vi "Calc_Average_Counts.vi"(0 "Mode":enum16{"Initialize", "Accumulate"}(ring), 2 "NumPixels":i32, 3 "Spectra":dbl[](array[numeric]), 5 "Pressure in":dbl, 6 "Temperature in":dbl, 7 "error in":errorcluster, 8 "State in":i32, 10 "Calculation config data":T1) -> (9 "First?":bool, 12 "Pressure during R":dbl, 14 "Temperature during R":dbl, 16 "R counts":dbl[](array[numeric]), 18 "Zero counts":dbl[](array[numeric]), 19 "Calc R?":bool, 20 "Ch1 Dark":dbl[](array[numeric]), 21 "Pressure during Zero":dbl, 22 "Temperature during Zero":dbl, 27 "error out":errorcluster)   [LabVIEW 2025]
uses:
  Configuration/TypeDef_CalculationConfigData.ctl
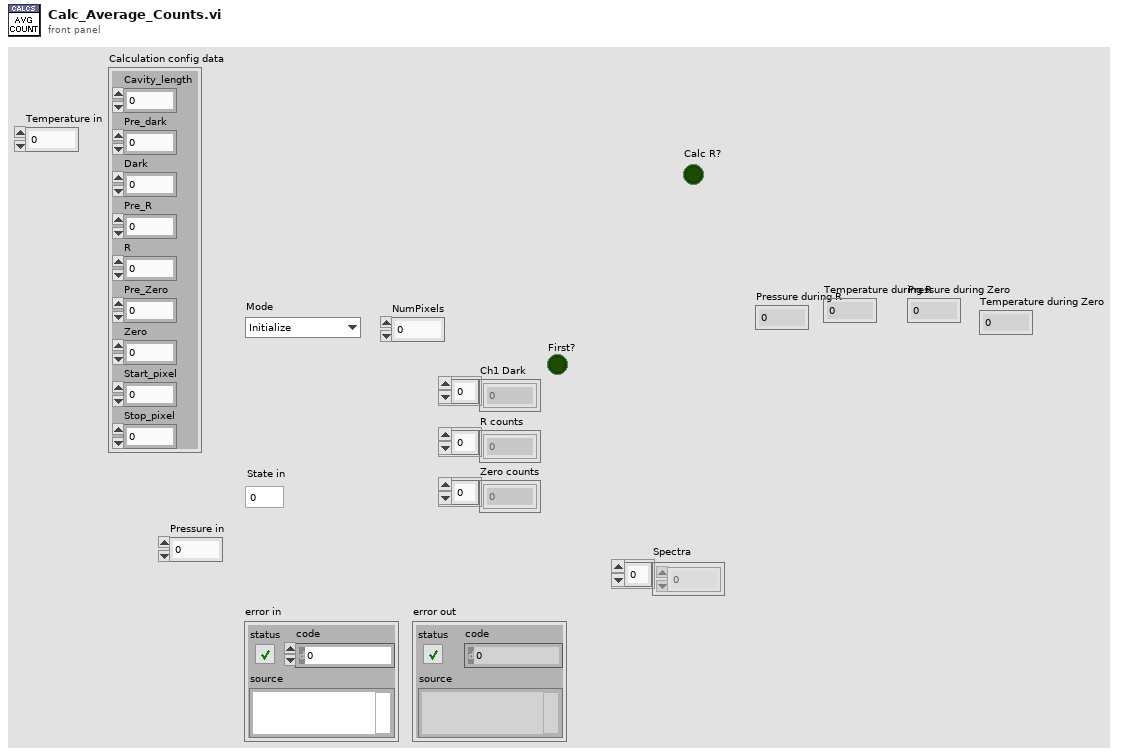
[diagram p1: front panel]
types:
  T1 = typedef "TypeDef_CalculationConfigData.ctl" = cluster{"Cavity_length":dbl, "Pre_dark":i32, "Dark":i32, "Pre_R":i32, "R":i32, "Pre_Zero":i32, "Zero":i32, "Start_pixel":i32, "Stop_pixel":i32}
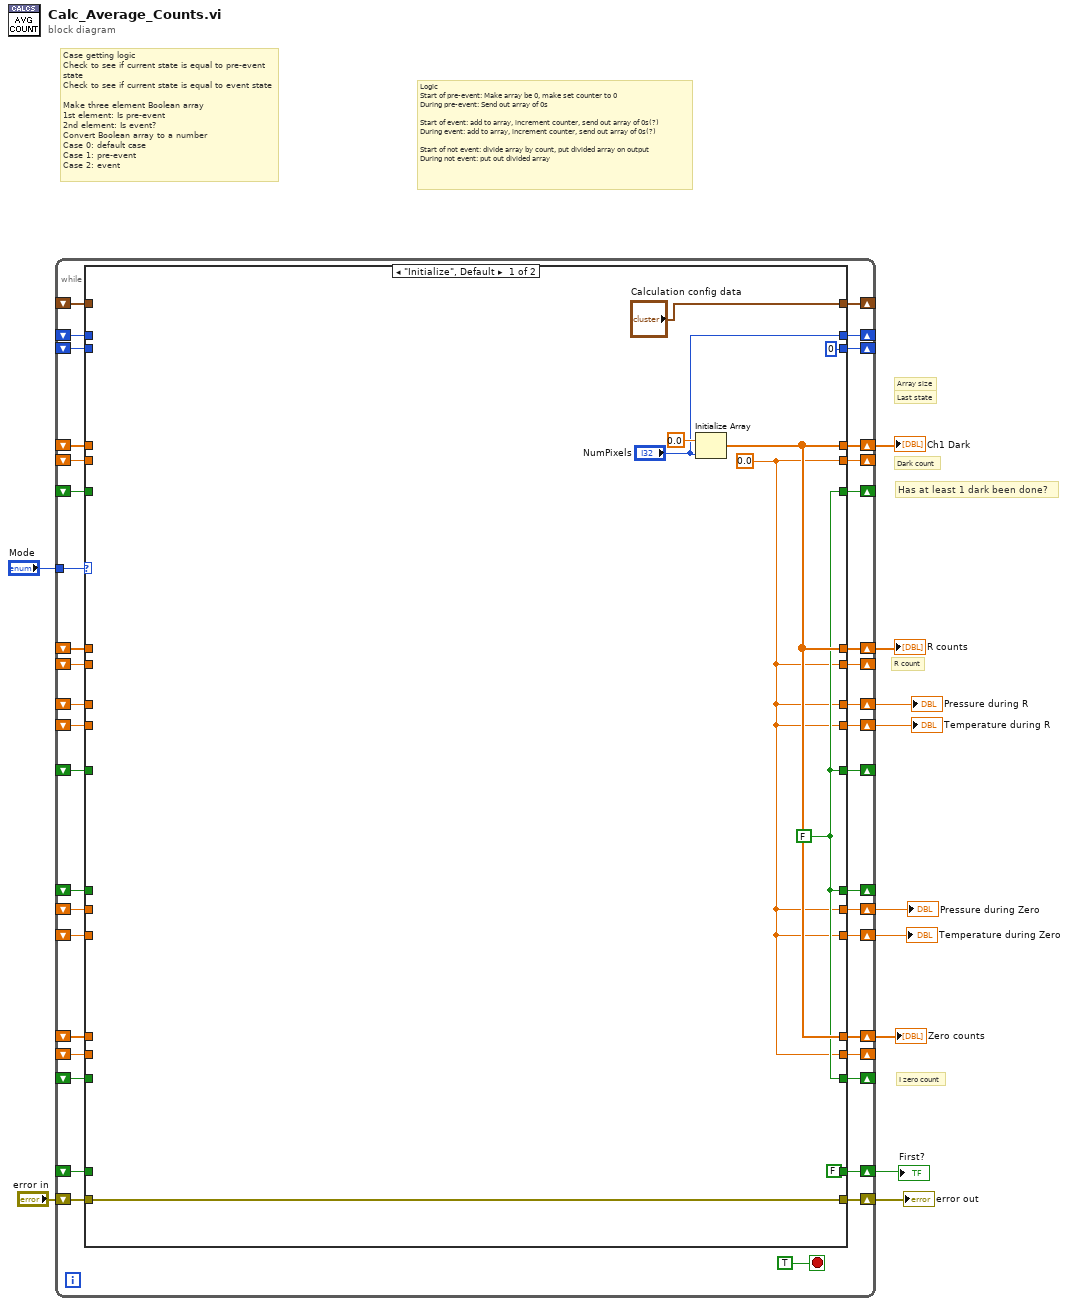
[diagram p0: block diagram]
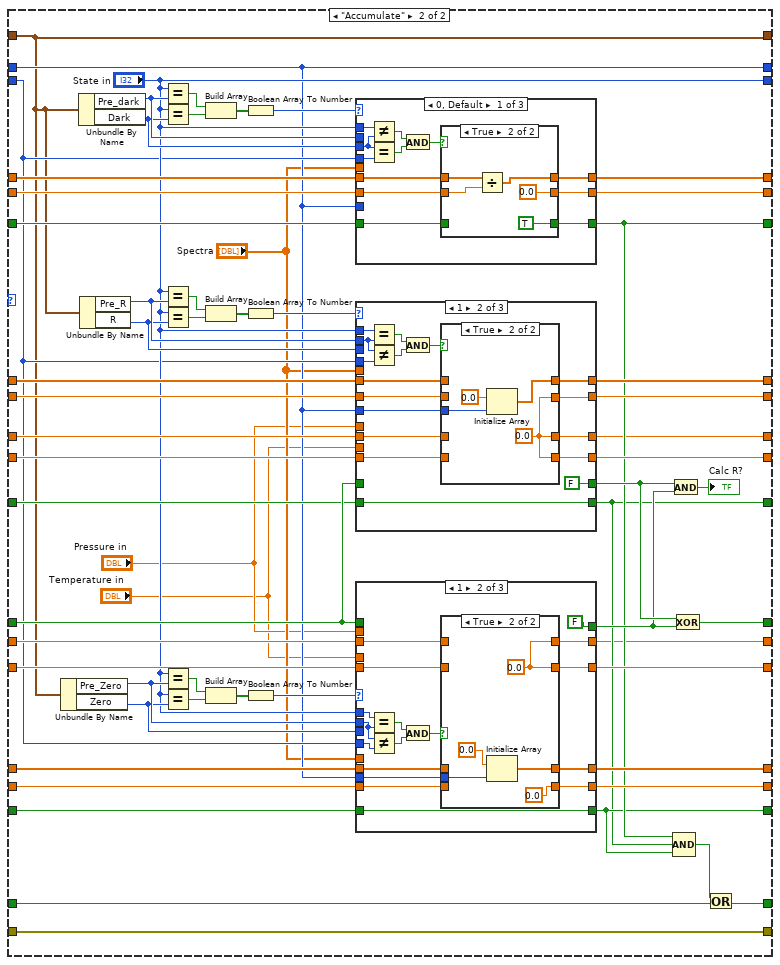
[diagram p2: hidden frame]
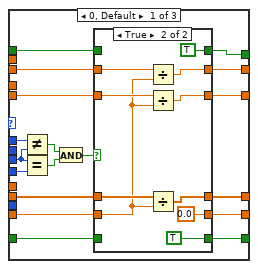
[diagram p3: hidden frame]
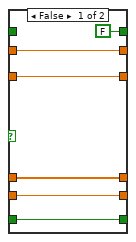
[diagram p4: hidden frame]
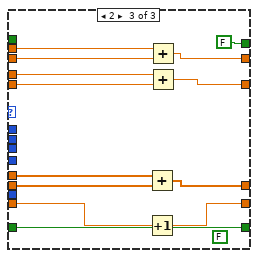
[diagram p6: hidden frame]
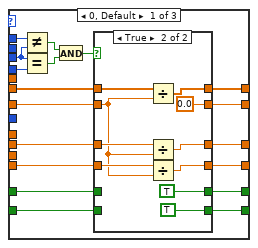
[diagram p7: hidden frame]
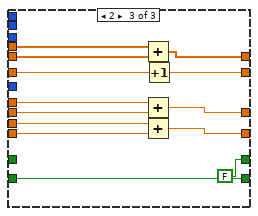
[diagram p10: hidden frame]
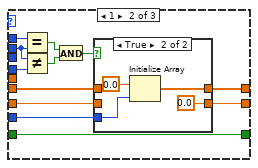
[diagram p12: hidden frame]
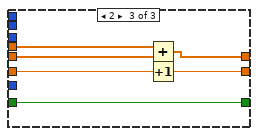
[diagram p14: hidden frame]
diagram:
  # "Has at least 1 dark been done?"
  # "Case getting logic\nCheck to see if current state is equal to pre-event state\nCheck to see if current state is equal to event state\n\nMake three element Boolean array \n1st element: Is pre-event\n2nd element: Is event?\nConvert Boolean array to a number\nCase 0: default case\nCase 1: pre-event\nCase 2: event"
  # "Logic\nStart of pre-event: Make array be 0, make set counter to 0\nDuring pre-event: Send out array of 0s\n\nStart of event: add to array, increment counter, send out array of 0s(?)\nDuring event: add to array, increment counter, send out array of 0s(?)\n\nStart of not event: divide array by count, put divided array on output\nDuring not event: put out divided array"
  # "Array size"
  # "Last state"
  # "I zero count"
  # "R count"
  # "Dark count"
  n1 = while {
    tunnel: "Mode" -> [w50]
    shift-right: [w48] -> w9
    shift-left: "error in" -> [w49]
    shift-right: [w47] -> w8
    shift-left: _ -> [w46]
    shift-right: [w45] -> _
    shift-left: _ -> [w34]
    shift-right: [w44] -> w7
    shift-left: _ -> [w42]
    shift-right: [w43] -> w6
    shift-left: _ -> [w41]
    shift-right: [w40] -> _
    shift-left: _ -> [w37]
    shift-right: [w39] -> _
    shift-left: _ -> [w38]
    shift-right: [w36] -> _
    shift-left: _ -> [w35]
    shift-right: [w33] -> _
    shift-left: _ -> [w32]
    shift-right: [w14] -> w2
    shift-left: _ -> [w28]
    shift-right: [w31] -> w1
    shift-left: _ -> [w27]
    shift-right: [w29] -> w4
    shift-left: _ -> [w26]
    shift-right: [w30] -> w3
    shift-left: _ -> [w25]
    shift-right: [w24] -> _
    shift-left: _ -> [w23]
    shift-right: [w22] -> w5
    shift-left: _ -> [w21]
    shift-right: [w20] -> _
    shift-left: _ -> [w16]
    shift-right: [w19] -> _
    shift-left: _ -> [w15]
    shift-right: [w18] -> _
    shift-left: _ -> [w17]
    shift-right: [w13] -> _
    shift-left: _ -> [w12]
    stop <- TRUE stop-if-true
    n2 = case shown="\"Initialize\", Default" w50 {
      tunnel: w49 -> [w60 w120]
      tunnel: [w60 w120] -> w48
      tunnel: [w56 w113] -> w47
      tunnel: w46 -> [_ w115]
      tunnel: [w53 w112] -> w45
      tunnel: [w56 w105] -> w44
      tunnel: [w56 w97] -> w43
      tunnel: w42 -> [_ w106]
      tunnel: w41 -> [_ w99]
      tunnel: [w53 w103] -> w40
      tunnel: [w53 w96] -> w39
      tunnel: w38 -> [_ w98]
      tunnel: w37 -> [_ w104]
      tunnel: [0 ("dimension size") "State in"] -> w36
      tunnel: w35 -> [_ w69]
      tunnel: w34 -> [_ w114]
      tunnel: ["NumPixels" w68] -> w33
      tunnel: w32 -> [_ w68]
      tunnel: [w53 w63] -> w14
      tunnel: [w53 w87] -> w31
      tunnel: [w53 w84] -> w30
      tunnel: [w53 w67] -> w29
      tunnel: w28 -> [_ w89]
      tunnel: w27 -> [_ w88]
      tunnel: w26 -> [_ w86]
      tunnel: w25 -> [_ w85]
      tunnel: [w54 w83] -> w24
      tunnel: w23 -> [_ w80]
      tunnel: [FALSE w77] -> w22
      tunnel: w21 -> [_ w78]
      tunnel: [w54 w76] -> w20
      tunnel: [w54 w72] -> w19
      tunnel: [w54 w73] -> w18
      tunnel: w17 -> [_ w74]
      tunnel: w16 -> [_ w75]
      tunnel: w15 -> [_ w71]
      tunnel: ["Calculation config data" w61] -> w13
      tunnel: w12 -> [_ w61]
      frame "Initialize", Default {
        w54 = FALSE
        w53 = 0.0 ("dimension size")
        n3 = Initialize Array(0.0 ("element"), "NumPixels") -> (w56:dbl[])
      }
      frame "Accumulate" {
        n4 = Unbundle By Name(w61) -> ("Pre_Zero"=w91:i32, "Zero"=w90:i32)
        n5 = Unbundle By Name(w61) -> ("Pre_dark"=w111:i32, "Dark"=w110:i32)
        n6 = Unbundle By Name(w61) -> ("Pre_R"=w101:i32, "R"=w100:i32)
        n7 = Equal?(x="State in", y=w111) -> (x = y?=w118:bool)
        n8 = Equal?(x="State in", y=w110) -> (x = y?=w119:bool)
        n9 = Equal?(x="State in", y=w101) -> (x = y?=w108:bool)
        n10 = Equal?(x="State in", y=w100) -> (x = y?=w107:bool)
        n11 = Equal?(x="State in", y=w91) -> (x = y?=w94:bool)
        n12 = Equal?(x="State in", y=w90) -> (x = y?=w95:bool)
        n13 = Build Array(w118, w119) -> (w117:bool[])
        n14 = Build Array(w108, w107) -> (w109:bool[])
        n15 = Build Array(w94, w95) -> (w93:bool[])
        n16 = Boolean Array To Number(Boolean array=w117) -> (number=w116:u32)
        n17 = Boolean Array To Number(Boolean array=w109) -> (number=w102:u32)
        n18 = Boolean Array To Number(Boolean array=w93) -> (number=w92:u32)
        n19 = case shown="0, Default" w116 {
          tunnel: w115 -> [w277 w294 w309]
          tunnel: w114 -> [w275 w293 w307]
          tunnel: "State in" -> [w273 w291 _]
          tunnel: w69 -> [w271 w292 _]
          tunnel: [w276 w296 w308] -> w113
          tunnel: [w274 w295 w306] -> w112
          tunnel: w68 -> [_ w297 _]
          tunnel: w111 -> [_ w290 _]
          tunnel: w110 -> [w272 _ _]
          tunnel: "Spectra" -> [_ _ w305]
          tunnel: [w267 w286 w304] -> w76
          tunnel: w75 -> [w266 w286 w304]
          frame 0, Default {
            n20 = Not Equal?(x=w273, y=w272) -> (x != y?=w269:bool)
            n21 = Equal?(x=w272, y=w271) -> (x = y?=w270:bool)
            n22 = And(x=w269, y=w270) -> (x .and. y?=w268:bool)
            n23 = case shown="True" w268 {
              tunnel: w277 -> [w280 w285]
              tunnel: [w280 w284] -> w276
              tunnel: w275 -> [w279 w282]
              tunnel: [w279 0.0 ("element")] -> w274
              tunnel: [w278 TRUE] -> w267
              tunnel: w266 -> [w278 _]
              frame False {
              }
              frame True {
                n24 = Divide(x=w285, y=w282) -> (x/y=w284:dbl[])
              }
            }
          }
          frame 1 {
            n25 = Equal?(x=w291, y=w290) -> (x = y?=w289:bool)
            n26 = Not Equal?(x=w290, y=w292) -> (x != y?=w288:bool)
            n27 = And(x=w289, y=w288) -> (x .and. y?=w287:bool)
            n28 = case shown="True" w287 {
              tunnel: w297 -> [_ w303]
              tunnel: [w299 w300] -> w296
              tunnel: [w298 0.0 ("element")] -> w295
              tunnel: w294 -> [w299 _]
              tunnel: w293 -> [w298 _]
              frame False {
              }
              frame True {
                n29 = Initialize Array(0.0 ("element"), w303) -> (w300:dbl[])
              }
            }
          }
          frame 2 {
            n30 = Add(x=w305, y=w309) -> (x+y=w308:dbl[])
            n31 = Increment(x=w307) -> (x+1=w306:dbl)
          }
        }
        n32 = case shown="1" w102 {
          tunnel: w106 -> [w211 w241 w265]
          tunnel: w104 -> [w209 w240 w263]
          tunnel: "State in" -> [w207 w238 _]
          tunnel: w69 -> [w205 w239 _]
          tunnel: [w210 w243 w264] -> w105
          tunnel: [w208 w242 w262] -> w103
          tunnel: w68 -> [_ w244 _]
          tunnel: w101 -> [_ w237 _]
          tunnel: w100 -> [w206 _ _]
          tunnel: "Spectra" -> [_ _ w261]
          tunnel: w89 -> [w201 w230 w253]
          tunnel: [w200 w232 w254] -> w63
          tunnel: w88 -> [w199 w233 w260]
          tunnel: [w198 w231 w259] -> w87
          tunnel: "Pressure in" -> [_ _ w258]
          tunnel: "Temperature in" -> [_ _ w257]
          tunnel: [w197 FALSE FALSE] -> w82
          tunnel: w80 -> [w196 _ _]
          tunnel: [w195 w229 w256] -> w72
          tunnel: w71 -> [w194 w229 w256]
          frame 0, Default {
            n33 = Not Equal?(x=w207, y=w206) -> (x != y?=w203:bool)
            n34 = Equal?(x=w206, y=w205) -> (x = y?=w204:bool)
            n35 = And(x=w203, y=w204) -> (x .and. y?=w202:bool)
            n36 = case shown="True" w202 {
              tunnel: w211 -> [w217 w227]
              tunnel: [w217 w226] -> w210
              tunnel: w209 -> [w216 w219]
              tunnel: [w216 0.0 ("element")] -> w208
              tunnel: w201 -> [w215 w224]
              tunnel: [w215 w223] -> w200
              tunnel: w199 -> [w214 w221]
              tunnel: [w214 w222] -> w198
              tunnel: [w213 TRUE] -> w197
              tunnel: w196 -> [w213 _]
              tunnel: [w212 TRUE] -> w195
              tunnel: w194 -> [w212 _]
              frame False {
              }
              frame True {
                n37 = Divide(x=w227, y=w219) -> (x/y=w226:dbl[])
                n38 = Divide(x=w224, y=w219) -> (x/y=w223:dbl)
                n39 = Divide(x=w221, y=w219) -> (x/y=w222:dbl)
              }
            }
          }
          frame 1 {
            n40 = Equal?(x=w238, y=w237) -> (x = y?=w236:bool)
            n41 = Not Equal?(x=w237, y=w239) -> (x != y?=w235:bool)
            n42 = And(x=w236, y=w235) -> (x .and. y?=w234:bool)
            n43 = case shown="True" w234 {
              tunnel: w244 -> [_ w252]
              tunnel: [w248 w250] -> w243
              tunnel: [w247 w249] -> w242
              tunnel: w241 -> [w248 _]
              tunnel: w240 -> [w247 _]
              tunnel: w233 -> [w246 _]
              tunnel: [w245 w249] -> w232
              tunnel: [w246 w249] -> w231
              tunnel: w230 -> [w245 _]
              frame False {
              }
              frame True {
                w249 = 0.0 ("element")
                n44 = Initialize Array(0.0 ("element"), w252) -> (w250:dbl[])
              }
            }
          }
          frame 2 {
            n45 = Add(x=w261, y=w265) -> (x+y=w264:dbl[])
            n46 = Add(x=w258, y=w253) -> (x+y=w254:dbl)
            n47 = Add(x=w257, y=w260) -> (x+y=w259:dbl)
            n48 = Increment(x=w263) -> (x+1=w262:dbl)
          }
        }
        n49 = case shown="1" w92 {
          tunnel: w99 -> [w138 w168 w193]
          tunnel: w98 -> [w136 w167 w191]
          tunnel: "State in" -> [w134 w165 _]
          tunnel: w69 -> [w132 w166 _]
          tunnel: [w137 w170 w192] -> w97
          tunnel: [w135 w169 w190] -> w96
          tunnel: w68 -> [_ w171 _]
          tunnel: w91 -> [_ w164 _]
          tunnel: w90 -> [w133 _ _]
          tunnel: "Spectra" -> [_ _ w189]
          tunnel: w86 -> [w128 w160 w188]
          tunnel: [w126 w159 w181] -> w67
          tunnel: "Pressure in" -> [_ _ w187]
          tunnel: "Temperature in" -> [_ _ w186]
          tunnel: w85 -> [w127 w155 w185]
          tunnel: [w125 w158 w184] -> w84
          tunnel: w80 -> [w124 _ _]
          tunnel: [w123 FALSE FALSE] -> w81
          tunnel: [w122 w156 w182] -> w73
          tunnel: w74 -> [w121 w156 w182]
          frame 0, Default {
            n50 = Not Equal?(x=w134, y=w133) -> (x != y?=w130:bool)
            n51 = Equal?(x=w133, y=w132) -> (x = y?=w131:bool)
            n52 = And(x=w130, y=w131) -> (x .and. y?=w129:bool)
            n53 = case shown="True" w129 {
              tunnel: w138 -> [w144 w154]
              tunnel: [w144 w153] -> w137
              tunnel: w136 -> [w143 w147]
              tunnel: [w143 0.0 ("element")] -> w135
              tunnel: w128 -> [w142 w151]
              tunnel: w127 -> [w141 w150]
              tunnel: [w142 w149] -> w126
              tunnel: [w141 w148] -> w125
              tunnel: [FALSE TRUE] -> w123
              tunnel: w124 -> [_ _]
              tunnel: [w139 TRUE] -> w122
              tunnel: w121 -> [w139 _]
              frame False {
              }
              frame True {
                n54 = Divide(x=w151, y=w147) -> (x/y=w149:dbl)
                n55 = Divide(x=w150, y=w147) -> (x/y=w148:dbl)
                n56 = Divide(x=w154, y=w147) -> (x/y=w153:dbl[])
              }
            }
          }
          frame 1 {
            n57 = Equal?(x=w165, y=w164) -> (x = y?=w163:bool)
            n58 = Not Equal?(x=w164, y=w166) -> (x != y?=w162:bool)
            n59 = And(x=w163, y=w162) -> (x .and. y?=w161:bool)
            n60 = case shown="True" w161 {
              tunnel: w171 -> [_ w180]
              tunnel: [w175 w177] -> w170
              tunnel: [w174 0.0 ("element")] -> w169
              tunnel: w168 -> [w175 _]
              tunnel: w167 -> [w174 _]
              tunnel: w160 -> [w173 _]
              tunnel: [w173 w176] -> w159
              tunnel: [w172 w176] -> w158
              tunnel: w155 -> [w172 _]
              frame False {
              }
              frame True {
                w176 = 0.0 ("element")
                n61 = Initialize Array(0.0 ("element"), w180) -> (w177:dbl[])
              }
            }
          }
          frame 2 {
            (unwired) FALSE
            n62 = Add(x=w189, y=w193) -> (x+y=w192:dbl[])
            n63 = Increment(x=w191) -> (x+1=w190:dbl)
            n64 = Add(x=w187, y=w188) -> (x+y=w181:dbl)
            n65 = Add(x=w186, y=w185) -> (x+y=w184:dbl)
          }
        }
        n66 = And(x=w82, y=w81) -> (x .and. y?=→"Calc R?":bool)
        n67 = Exclusive Or(1:w81, 2:w82) -> (0:w83:bool)
        n68 = Compound Arithmetic op=AND(w76, w72, w73) -> (w79:bool)
        n69 = Or(x=w79, y=w78) -> (x .or. y?=w77:bool)
      }
    }
  }
  "error out" <- w9
  "Ch1 Dark" <- w8
  "R counts" <- w7
  "Zero counts" <- w6
  "Pressure during R" <- w2
  "Temperature during R" <- w1
  "Pressure during Zero" <- w4
  "Temperature during Zero" <- w3
  "First?" <- w5
